vi "Digital Debounce Filter.vi"(0 "Boolean input":bool, 1 "Error In":errorcluster) -> (2 "Rising Edge":bool, 3 "A/DIO0 presses":i32, 4 "Error Out":errorcluster)   [LabVIEW 2018]
uses:
  <vilib>/ErrorRing/Error Ring.xnode
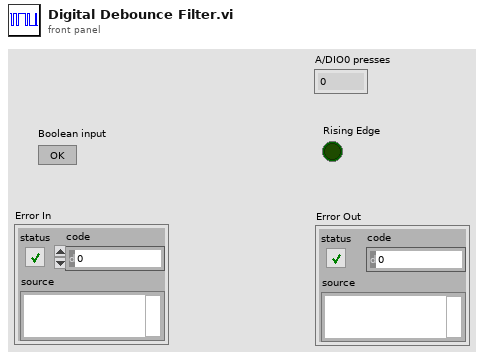
[diagram p1: front panel]
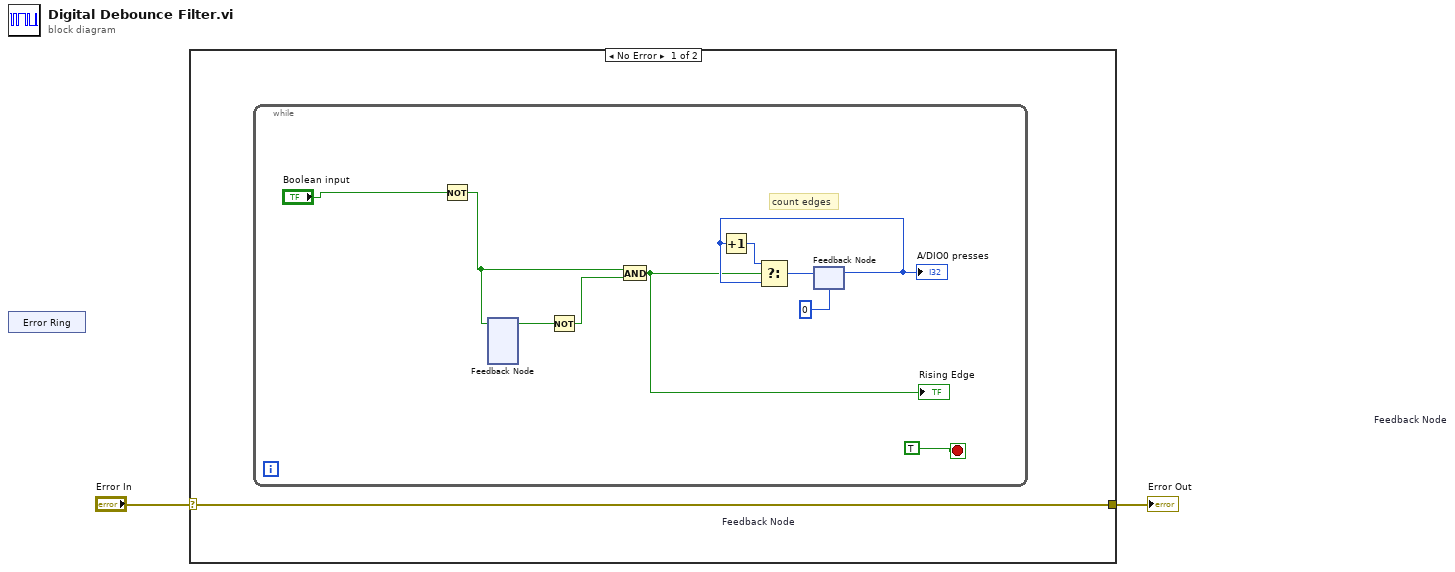
[diagram p0: block diagram]
diagram:
  n1 = xnode "Error Ring"() -> ()  [unwired: 1 out]
  n2 = case shown="No Error" "Error In" {
    selector: "Error In" -> [w3 w14]
    tunnel: [w3 w14] -> w1
    frame No Error {
      n3 = while {
        stop <- TRUE ("stop") stop-if-true
        # "count edges"
        n4 = Not(x="Boolean input") -> (.not. x?=w10:bool)
        n5 = feedback #1 "Feedback Node"() -> (w9:bool)  [unwired: 1 in]
        n6 = feedback-in #1(w10) -> ()
        n7 = Not(x=w9) -> (.not. x?=w13:bool)
        n8 = And(x=w10, y=w13) -> (x .and. y?=w4:bool)
        "Rising Edge" <- w4
        n9 = feedback #2 "Feedback Node"(0) -> (w5:i32)
        "A/DIO0 presses" <- w5
        n10 = Increment(x=w5) -> (x+1=w7:i32)
        n11 = Select(t=w7, s=w4, f=w5) -> (s? t:f=w6:i32)
        n12 = feedback-in #2(w6) -> ()
      }
    }
    frame Error {
    }
  }
  "Error Out" <- w1
